vi "Measure Sound from Digital Mic - I2S.vi"() -> ()   [LabVIEW 2022 SP3]
doc: "This example performs a continuous acquisition of PCM data. At the same time, the GPIO lines are used for digital input and digital output."
uses:
  <vilib>/PDM Acquisition Toolkit/host/Classes/Session/Controls/Logic Levels.ctl
  <vilib>/PDM Acquisition Toolkit/shared/controls/PCM Data Format Configuration.ctl
  <vilib>/PDM Acquisition Toolkit/shared/controls/Digital Edge.ctl
  <vilib>/PDM Acquisition Toolkit/shared/controls/PCM Bit Endianness.ctl
  <vilib>/PDM Acquisition Toolkit/shared/controls/PCM Data Justification.ctl
  <vilib>/PDM Acquisition Toolkit/host/Classes/Tasks/PDM Tasks/Controls/Acquisition Mode.ctl
  <vilib>/PDM Acquisition Toolkit/shared/controls/clock mode.ctl
  <vilib>/PDM Acquisition Toolkit/shared/controls/PCM Frame Sync Control.ctl
  <vilib>/addons/_NISVFA/_Shared subVIs/Common/SVL Set dB Reference (1 Ch).vi
  <vilib>/addons/Sound and Vibration/svt_Level/SVL AC & DC Level (Time) (1 Ch).vi
  <vilib>/addons/_NISVFA/_Shared subVIs/Common/SVL Set dB Reference (variant).vi
  <vilib>/addons/_NISVFA/_Shared subVIs/Common/svc_Get SV Channel Info.vi
  <vilib>/Analysis/baseanly.llb/Mean.vi
  <vilib>/Analysis/baseanly.llb/Mean (DBL).vi
  <vilib>/addons/_NISVFA/_Shared subVIs/Windowing/svfa_Scaled Time Domain Window (Array).vi
  <vilib>/addons/_NISVFA/_Shared subVIs/Common/svc_Unit Label to Engineering Units.vi
  <vilib>/addons/_NISVFA/_Shared subVIs/Common/svc_Engineering Units to Unit Label.vi
  <vilib>/addons/_NISVFA/_Spectrum Processing/subVIs/svfa_Spectrum Info Window to windowTd Type Def.vi
  <vilib>/Analysis/4window.llb/Force Window.vi
  <vilib>/Analysis/4window.llb/Force Window (DBL).vi
  <vilib>/Analysis/4window.llb/Exponential Window.vi
  <vilib>/Analysis/4window.llb/Exponential Window (DBL).vi
  <vilib>/PDM Acquisition Toolkit/host/API/Public/Create Tasks/Create PCM Input Task.vi
  <vilib>/PDM Acquisition Toolkit/host/API/Public/Configure/Timing/Configure Timing - PCM Input Master.vi
  <vilib>/PDM Acquisition Toolkit/host/API/Public/Configure/PDM Channel/Configure Microphone Sensitivity DBFS - PCM Input Task.vi
  <vilib>/PDM Acquisition Toolkit/host/API/Public/Start/Start PCM Input Task.vi
  <vilib>/PDM Acquisition Toolkit/host/API/Public/Read/Read PCM Input Waveform.vi
  <vilib>/addons/_NISVFA/_Shared subVIs/Common/svc_Caller VI Returned in Error Source.vi
  <vilib>/addons/_NISVFA/_Shared subVIs/Common/svc_Get Window Info.vi
  <vilib>/Analysis/0measdsp.llb/Scaled Time Domain Window.vi
  <vilib>/Analysis/0measdsp.llb/Scaled Time Domain Window (DBL).vi
  <vilib>/Utility/error.llb/Error Cluster From Error Code.vi
  <vilib>/Analysis/baseanly.llb/Std Deviation and Variance.vi
  <vilib>/addons/Sound and Vibration/svt_Weighting/SVT Weighting Filter (1 Ch).vi
  <vilib>/addons/Sound and Vibration/svt_Level/SVL Leq Sound Level (1 Ch).vi
  <vilib>/PDM Acquisition Toolkit/host/API/Public/Stop/Stop PCM Input Task.vi
  <vilib>/PDM Acquisition Toolkit/host/API/Public/Clear/Clear PCM Input Task.vi
  <vilib>/PDM Acquisition Toolkit/host/API/PDM Acquisition Toolkit.lvlib
  <vilib>/PDM Acquisition Toolkit/host/Classes/Tasks/PDM Tasks/PDM Task.lvclass
  <vilib>/PDM Acquisition Toolkit/shared/PDM Shared.lvlib
  <vilib>/addons/Sound and Vibration/svt_Weighting/SoundVib_ABCWeighting.lvlib
  <vilib>/addons/Sound and Vibration/svt_Level/SoundVib_SoundLevel.lvlib
  <vilib>/PDM Acquisition Toolkit/host/Classes/Session/DecoderSession.lvclass
panel:
  out "Leq sound level [dB EU]":dbl=93.30183477798138 format="%.2f"
  in  "weighting":u16(ring) items=["Linear", "A-weighting", "B-weighting", "C-weighting"]
  in  "PCM data configuration":T1={"Frame Sync Edge for Channel 0"=enum."Falling", "Channel Count Per Frame"=2, "Channel Length"=32, "Bit Depth"=24, "Channel 0 Offset"=1, "Endianness"=enum."MSB First", "Data Justification"=enum."Left Justified"}
  out "actual Bit Clock rate":sgl=3200000.0 format="%.5p"
  out "Error Out":errorcluster
  out "Waveform Graph":waveform(dbl)(graph)={"t0"=timestamp(0 s since 1904-01-01), "dt"=1.9999999494757503e-05, "Y"=[], "attributes"=variant("NI_ChannelName"=variant(string "PCMI8.0"), "NI_dBReference"=variant(dbl 2e-05))}
  in  "Number of Samples":i32=10000
  in  "I2S Channels":string="PXI1Slot5\\PCMi 8"
  in  "Logic Level":T5
  in  "Microphone Sensitivity (dBFS)":dbl=-26.0 format="%#_13g"
  in  "Stop":bool
  # "PDM Input"
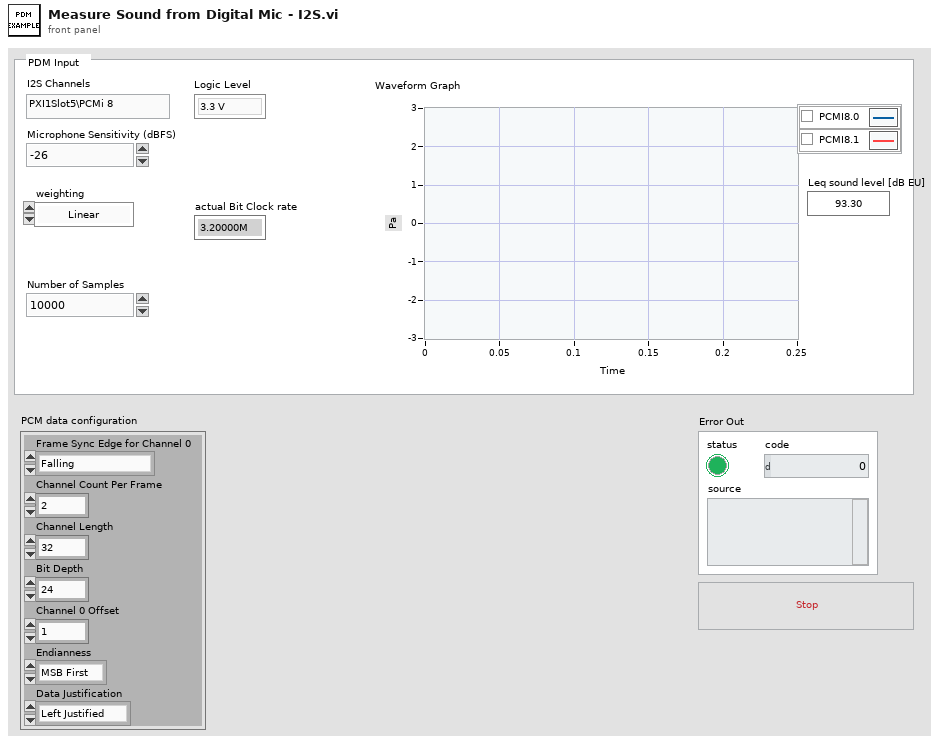
[diagram p1: front panel]
types:
  T1 = typedef "PDM Shared.lvlib/PCM Data Format Configuration.ctl" = cluster{"Frame Sync Edge for Channel 0":T2, "Channel Count Per Frame":u8, "Channel Length":u16, "Bit Depth":u8, "Channel 0 Offset":u16, "Endianness":T3, "Data Justification":T4}
  T2 = typedef "PDM Shared.lvlib/Digital Edge.ctl" = enum8{"Rising", "Falling"}
  T3 = typedef "PDM Shared.lvlib/PCM Bit Endianness.ctl" = enum16{"MSB First", "LSB First"}
  T4 = typedef "PDM Shared.lvlib/PCM Data Justification.ctl" = enum16{"Left Justified", "Right Justified"}
  T5 = typedef "PDM Acquisition Class Library.lvlib/DecoderSession.lvclass/Logic Levels.ctl" = enum16{"3.3 V", "1.8 V", "1.2 V"}
  T6 = typedef "PDM Shared.lvlib/PCM Frame Sync Control.ctl" = cluster{"Frame Length":u16, "Frame Sync Pulse Width":u16, "Bit Clock Edge  Sync":T2}
  T7 = typedef "PDM Shared.lvlib/clock mode.ctl" = enum16{"divided clock", "DDS"}
  T8 = typedef "PDM Acquisition Class Library.lvlib/PDM Task.lvclass/Acquisition Mode.ctl" = enum16{"Finite", "Continuous"}
  T9 = typedef "PDM Acquisition Class Library.lvlib/PCM Input Task.lvclass/DVR PCM Input Task.ctl" = refnum<data-value>
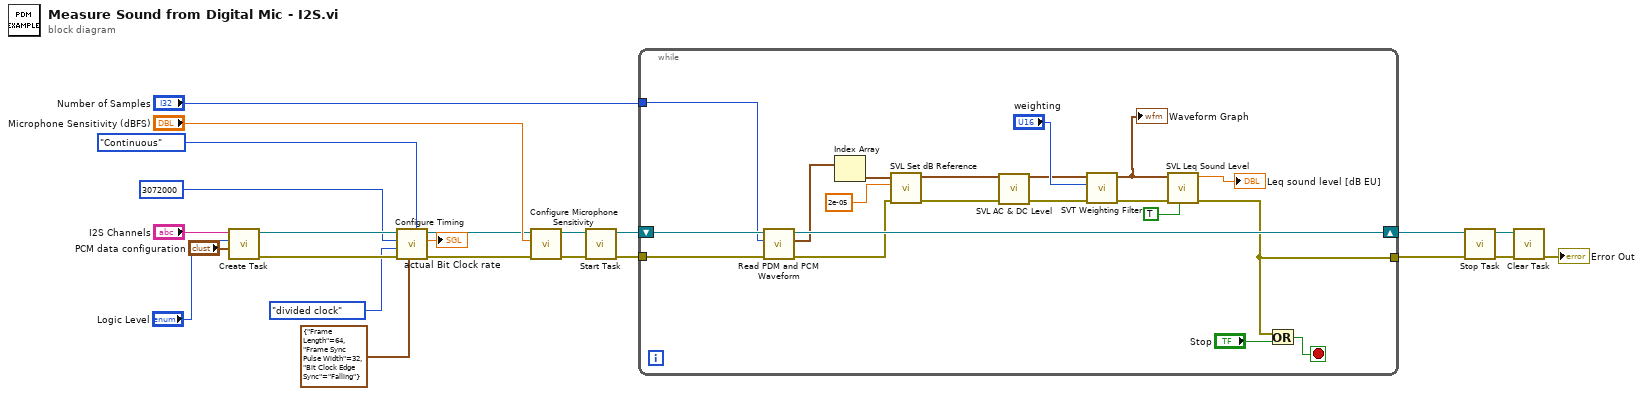
[diagram p0: block diagram]
diagram:
  n1 = call-poly <vilib>:"Create Task.vi"("PCM data configuration"="PCM data configuration", "logic level"="Logic Level", "channel list"="I2S Channels") -> ("error out"=w14:errorcluster, "PCM input task out"=w15:T9)  [unwired: 7 in]
  n2 = call-poly <vilib>:"Configure Timing.vi"("acquisition mode"=Acquisition_Mode."Continuous" ("Acquisition Mode"), "Frame Sync Clock Control"=T6 {"Frame Length"=64, "Frame Sync Pulse Width"=32, "Bit Clock Edge  Sync"=enum."Falling"}, "error in"=w14, "clock mode"=clock_mode."divided clock", "Bit Clock rate"=u32 3072000, "PCM input task in"=w15) -> ("error out"=w17:errorcluster, "actual Bit Clock rate"=→"actual Bit Clock rate":sgl, "PCM input task out"=w18:T9)  [unwired: 3 in]
  n3 = call-poly <vilib>:"Configure Microphone Sensitivity.vi"("error in"=w17, "microphone sensitivity (dBFS)"="Microphone Sensitivity (dBFS)", "PCM input task in"=w18) -> ("error out"=w11:errorcluster, "PCM input task out"=w10:T9)  [unwired: 7 in]
  n4 = call-poly <vilib>:"Start Task.vi"("error in"=w11, "PCM input task in"=w10) -> ("error out"=w8:errorcluster, "PCM input task out"=w9:T9)  [unwired: 8 in]
  n5 = while {
    tunnel: w8 -> [w40]
    tunnel: "Number of Samples" -> [w39]
    shift-right: [w42] -> w22
    shift-left: w9 -> [w41]
    tunnel: [w24] -> w1
    stop <- w38 stop-if-true
    n6 = call-poly <vilib>:"Read PDM and PCM Waveform.vi"("error in"=w40, "words per channel"=w39, "PCM input task In"=w41) -> ("error out"=w29:errorcluster, "PCM waveforms"=w30:waveform(dbl)[], "PCM input task out"=w42:T9)  [unwired: 3 in, 3 out]
    n7 = Index Array(array=w30) -> (element=w33:waveform(dbl))  [unwired: 1 in]
    n8 = call-poly <vilib>:"SVL Set dB Reference.vi"("error in (no error)"=w29, "dB reference [EU]"=2e-05, "scaled signal in [EU]"=w33) -> ("error out"=w32:errorcluster, "scaled signal out [EU]"=w26:waveform(dbl))  [unwired: 7 in]
    n9 = call-poly <vilib>:"SVL AC & DC Level.vi"("scaled signal [EU]"=w26) -> ("AC signal [EU]"=w25:waveform(dbl))  [unwired: 13 in, 5 out]
    n10 = call-poly <vilib>:"SVT Weighting Filter.vi"("error in (no error)"=w32, "weighting"="weighting", "scaled signal [EU]"=w25) -> ("error out"=w35:errorcluster, "weighted signal [EU]"=w28:waveform(dbl))  [unwired: 6 in]
    "Waveform Graph" <- w28
    n11 = call-poly <vilib>:"SVL Leq Sound Level.vi"("restart averaging (F)"=TRUE, "error in (no error)"=w35, "scaled signal [EU]"=w28) -> ("error out"=w24:errorcluster, "Leq sound level [dB EU]"=→"Leq sound level [dB EU]":dbl)  [unwired: 6 in, 1 out]
    n12 = Or(x=w24, y="Stop") -> (x .or. y?=w38:bool)
  }
  n13 = call-poly <vilib>:"Stop Task.vi"("error in"=w1, "PCM input task In"=w22) -> ("error out"=w16:errorcluster, "PCM input task out"=w21:T9)  [unwired: 8 in]
  n14 = call-poly <vilib>:"Clear Task.vi"("error in"=w16, "PCM input task in"=w21) -> ("error out"=→"Error Out":errorcluster)  [unwired: 9 in]
